vi "Splash Screen.vi"(9 "Skip Fade & Show Title Bar? (F)":bool) -> ()   [LabVIEW 2015]
doc: "*-----------------------------------------------------\n* Author: Swatts\n*\n* VI Description: Pops up the About box hello\n* \n*\n* Error handling: All errors passed out\n*\n* Pre-condition: \n*\n* Post-condition: None\n*\n* Revision History:\n*\n* Rev Date Author Description \n* 01 29/04/2014 SWatts First issue\n*\n*-----------------------------------------------------"
uses:
  <vilib>/Platform/browser.llb/Open URL in Default Browser (string).vi
panel:
  in  "Website":bool
  out "Version:":string
  # "Copyright 2011, Your Company, Inc.  IMAQ, LabVIEW, and NI-MAX are all registered trademarks of National Instruments (NI) in the US and other countries and are used with permission. All other product and brand names used in this document may be trademarks or registered trademarks of their respective owners in the US and/or in other countries."
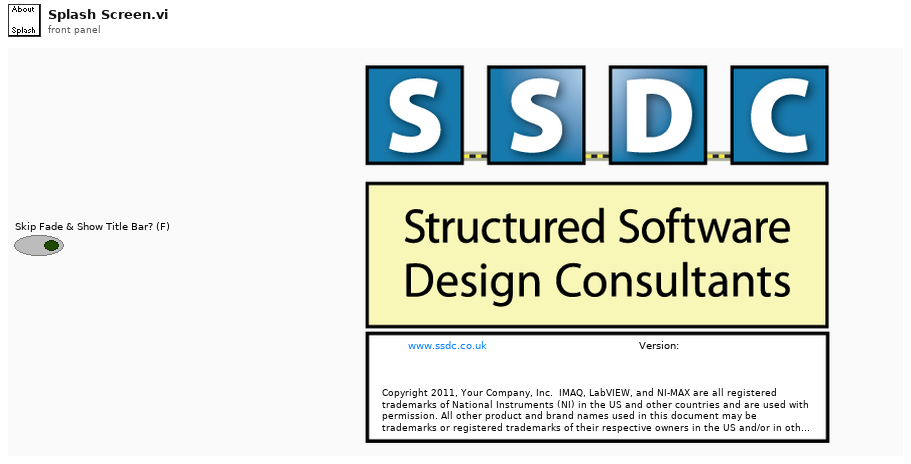
[diagram p1: front panel]
types:
  T1 = enum32{"Invalid", "Standard", "Closed", "Hidden", "Minimized", "Maximized"}
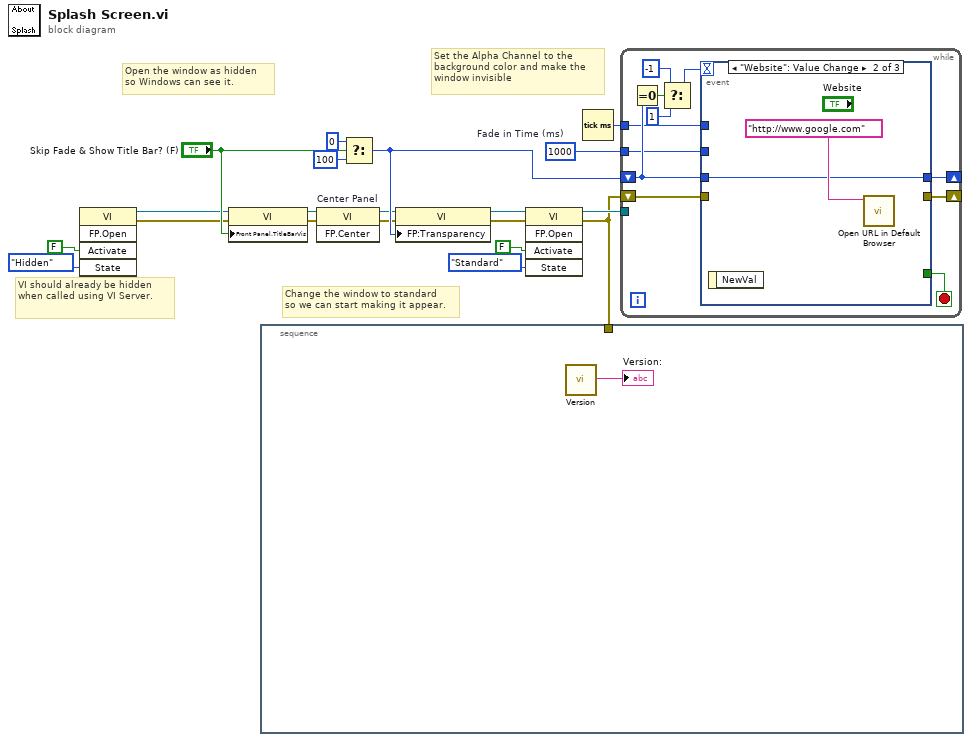
[diagram p0: block diagram]
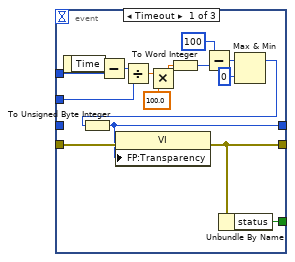
[diagram p2: hidden frame]
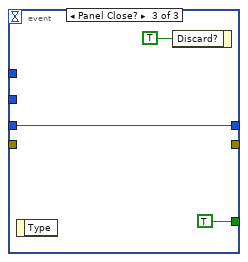
[diagram p3: hidden frame]
diagram:
  w14 = i16 1000  # Fade in Time (ms)
  # "VI should already be hidden when called using VI Server."
  # "Change the window to standard\nso we can start making it appear."
  # "Set the Alpha Channel to the\nbackground color and make the\nwindow invisible"
  # "Open the window as hidden\nso Windows can see it."
  n1 = invoke class="VI" method="FP.Open"("Activate"=FALSE ("Activate?"), "State"=T1."Hidden") -> (reference out=w5:refnum<vi>, error out=w1:errorcluster)  [unwired: 3 in, 3 out]
  n2 = property class="VI"(reference=w5, error in=w1, "Front Panel.TitleBarVis"="Skip Fade & Show Title Bar? (F)") -> (reference out=w4:refnum<vi>, error out=w8:errorcluster)
  n3 = invoke on="Center Panel" class="VI" method="FP.Center"(reference=w4, error in=w8) -> (reference out=w3:refnum<vi>, error out=w9:errorcluster)  [unwired: 1 in, 1 out]
  n4 = Select(t=u8 0, s="Skip Fade & Show Title Bar? (F)", f=u8 100 ("Factor")) -> (s? t:f=w11:u8)
  n5 = property class="VI"(reference=w3, error in=w9, "FP:Transparency"=w11) -> (reference out=w2:refnum<vi>, error out=w6:errorcluster)
  n6 = invoke class="VI" method="FP.Open"(reference=w2, error in=w6, "Activate"=FALSE ("Activate?"), "State"=T1."Standard") -> (reference out=w18:refnum<vi>, error out=w7:errorcluster)  [unwired: 1 in, 3 out]
  n7 = stacked-sequence {
    tunnel: w7 -> [_]
    frame #0 {
      n8 = call "Version.vi"() -> ("Version"=→"Version:":string)  [unwired: 5 in]
    }
  }
  n9 = Tick Count (ms)() -> (millisecond timer value=w15:u32)
  n10 = while {
    shift-right: [w32] -> _
    shift-left: w11 -> [w28]
    shift-right: [w30] -> _
    shift-left: w7 -> [w31]
    tunnel: w18 -> [_]
    tunnel: w15 -> [w23]
    tunnel: w14 -> [w22]
    stop <- w29 stop-if-true
    n11 = Equal To 0?(x=w28) -> (x = 0?=w27:bool)
    n12 = Select(t=-1, s=w27, f=1) -> (s? t:f=w24:i32)
    n13 = event shown="[1] \"Website\": Value Change" {
      selector: _ -> [_ _ _]
      dyn-events: _ -> [_ _ _]
      timeout: w24 -> [_ _ _]
      tunnel: w28 -> [_ w49 w51]
      tunnel: [w38 w49 w51] -> w32
      tunnel: w31 -> [w48 _ _]
      tunnel: [w47 _ _] -> w30
      tunnel: [w46 _ TRUE ("Close")] -> w29
      tunnel: w23 -> [w44 _ _]
      tunnel: w22 -> [w37 _ _]
      event Timeout {
        n14 = event-data() -> ("Time"=w45:u32)  [unwired: 1 in]
        n15 = Subtract(x=w45, y=w44) -> (x-y=w42:u32)
        n16 = Divide(x=w42, y=w37) -> (x/y=w35:dbl)
        n17 = Multiply(x=w35, y=100.0) -> (x*y=w33:dbl)
        n18 = To Word Integer(number=w33) -> (16bit integer=w39:i16)
        n19 = Subtract(x=i16 100 ("Factor"), y=w39) -> (x-y=w41:i16)
        n20 = Max & Min(x=w41, y=i16 0) -> (max(x,y)=w36:i16)  [unwired: 1 out]
        n21 = To Unsigned Byte Integer(number=w36) -> (unsigned 8bit integer=w38:u8)
        n22 = property class="VI"(error in=w48, "FP:Transparency"=w38) -> (error out=w47:errorcluster)  [unwired: 1 in, 1 out]
        n23 = Unbundle By Name(w47) -> ("status"=w46:bool)
      }
      event "Website": Value Change {
        n24 = event-data() -> ()  [unwired: 1 in, 1 out]
        n25 = call-poly <vilib>:"Open URL in Default Browser.vi"("URL"="http://www.google.com" ("Link")) -> ()  [unwired: 5 in, 2 out]
      }
      event Panel Close? {
        n26 = event-data() -> ()  [unwired: 1 in, 1 out]
        n27 = event-data("Discard?"=TRUE) -> ()  [unwired: 1 in, 1 out]
      }
    }
  }
